vi "NanMean.vi"(11 "Array":dbl[](array[numeric])) -> (3 "Nanmean":dbl)   [LabVIEW 2013]
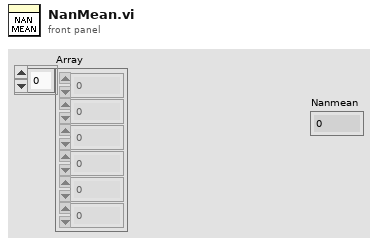
[diagram p1: front panel]
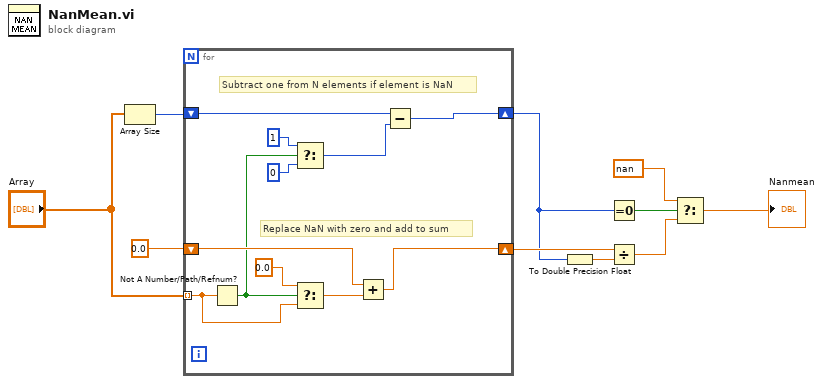
[diagram p0: block diagram]
diagram:
  n1 = Array Size(array="Array") -> (size(s)=w9:i32)
  n2 = for {
    tunnel: "Array" -> [w20] mode=indexing
    shift-right: [w17] -> w5
    shift-left: 0.0 -> [w18]
    shift-right: [w11] -> w3
    shift-left: w9 -> [w13]
    # "Replace NaN with zero and add to sum"
    # "Subtract one from N elements if element is NaN"
    n3 = Not A Number/Path/Refnum?(number/path/refnum=w20) -> (NaN/Path/Refnum?=w16:bool)
    n4 = Select(t=1, s=w16, f=0) -> (s? t:f=w12:i32)
    n5 = Select(t=0.0, s=w16, f=w20) -> (s? t:f=w19:dbl)
    n6 = Add(x=w18, y=w19) -> (x+y=w17:dbl)
    n7 = Subtract(x=w13, y=w12) -> (x-y=w11:i32)
  }
  n8 = To Double Precision Float(number=w3) -> (double precision float=w2:dbl)
  n9 = Equal To 0?(x=w3) -> (x = 0?=w7:bool)
  n10 = Divide(x=w5, y=w2) -> (x/y=w4:dbl)
  n11 = Select(t=nan, s=w7, f=w4) -> (s? t:f=→"Nanmean":dbl)
